vi "Connect.vi"(8 "error in (no error)":errorcluster, 10 "Session - Pipeline":path=path "Z:/users/Manolis/Labview/Cajal/Cajal-manolis.dsn", 11 "Database in":refnum<class "Database.lvclass">) -> (0 "error out":errorcluster, 3 "Database out":refnum<class "Database.lvclass">)   [LabVIEW 2014, in "Database.lvclass"]
uses:
  Database.lvclass
  <vilib>/addons/database/NI_Database_API.lvlib
  <vilib>/addons/database/Connection.llb/DB Tools Open Connec (Path).vi
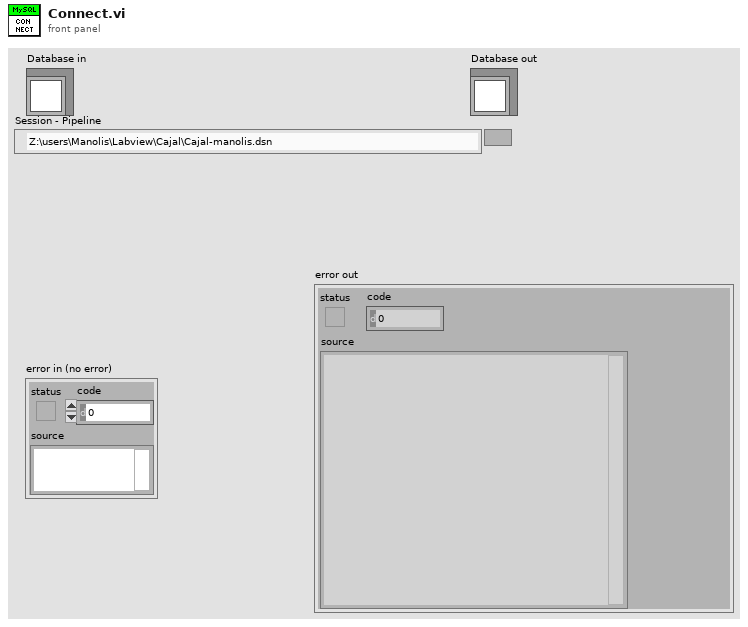
[diagram p1: front panel]
types:
  T1 = typedef "NI_Database_API.lvlib/Conn ObjectReference.ctl" = refnum<k1>
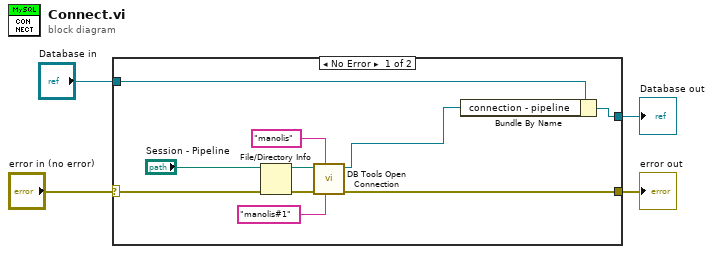
[diagram p0: block diagram]
diagram:
  n1 = case shown="No Error" "error in (no error)" {
    selector: "error in (no error)" -> [w9 w16]
    tunnel: [w5 w16] -> w3
    tunnel: [w13 w15] -> w1
    tunnel: "Database in" -> [w14 w15]
    frame No Error {
      n2 = File/Directory Info(path="Session - Pipeline", error in=w9) -> (path out=w11:path, error out=w8:errorcluster)  [unwired: 5 out]
      n3 = call-poly <vilib>:"DB Tools Open Connection.vi"("password"="manolis#1", "userID"="manolis", "error in (no error)"=w8, "connection information"=w11) -> ("error out"=w5:errorcluster, "connection reference"=w10:T1)  [unwired: 4 in]
      n4 = Bundle By Name(cluster=w14, "connection - pipeline"=w10) -> (w13:refnum<class "Database.lvclass">)
    }
    frame Error {
    }
  }
  "error out" <- w3
  "Database out" <- w1
